vi "__Update Bucket List.vi"(8 "error in (no error)":errorcluster, 11 "FileManager Ctl Refs in":T1) -> (0 "error out":errorcluster, 3 "FileManager Ctl Refs out":T1)   [LabVIEW 2011]
doc: "Requests the buckets owned by the user from Amazon S3 and then populates the Buckets ComboBox on the application front panel with the values."
uses:
  __File manager Data type.ctl
  vi.lib/National Instruments/LabVIEW Interface for Amazon S3/LV Interface for Amazon S3.lvlib
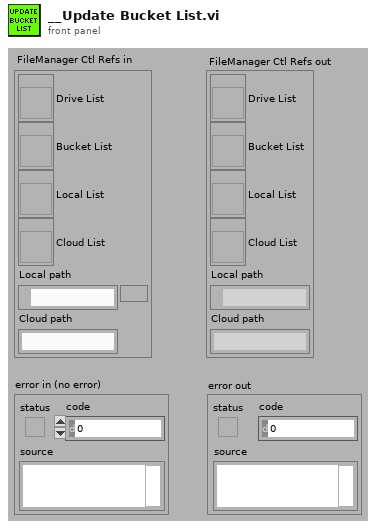
[diagram p1: front panel]
types:
  T1 = typedef "__File manager Data type.ctl" = cluster{"Drive List":refnum<vi>, "Bucket List":refnum<vi>, "Local List":refnum<vi>, "Cloud List":refnum<vi>, "Local path":path, "Cloud path":string}
  T2 = typedef "LV Interface for Amazon S3.lvlib/AMZ_S3_API_Bucket.ctl" = cluster{"Name":string, "CreationDate":timestamp}
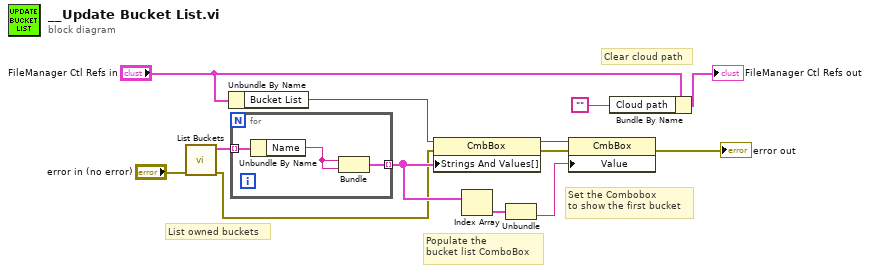
[diagram p0: block diagram]
diagram:
  # "Clear cloud path"
  # "Set the Combobox\nto show the first bucket"
  # "Populate the\nbucket list ComboBox"
  # "List owned buckets"
  n1 = call "List Buckets.vi"("error in (no error)"="error in (no error)") -> ("error out"=w4:errorcluster, "Buckets"=w5:T2[])  [unwired: 9 in]
  n2 = Unbundle By Name("FileManager Ctl Refs in") -> ("Bucket List"=w7:refnum<vi>)
  n3 = for {
    tunnel: [w16] -> w10 mode=indexing
    tunnel: w5 -> [w15] mode=indexing
    n4 = Unbundle By Name(w15) -> ("Name"=w14:string)
    n5 = Bundle("Name"=w14, "Name"=w14) -> (w16:cluster{"Name":string, "Name":string})  [unwired: 1 in]
  }
  n6 = property class="CmbBox"(reference=w7, error in=w4, "Strings And Values[]"=w10) -> (reference out=w11:refnum<vi>, error out=w12:errorcluster)
  n7 = Index Array(array=w10) -> (element=w9:cluster{"Name":string, "Name":string})  [unwired: 1 in]
  n8 = Unbundle(w9) -> ("Name"=w8:string)  [unwired: 1 out]
  n9 = property class="CmbBox"(reference=w11, error in=w12, "Value"=w8) -> (error out=→"error out":errorcluster)  [unwired: 1 out]
  n10 = Bundle By Name(cluster="FileManager Ctl Refs in", "Cloud path"="") -> (→"FileManager Ctl Refs out":T1)
